vi "Seconds_to_Elapsed_Time_String.vi"(10 "# Seconds (0)":u32) -> (2 "Elapsed Time (00:00:00)":string="00:00:00")   [LabVIEW 2014, in "UI_ProgressDlg.lvlib" / "UI_ProgressDlg.lvclass"]
doc: "This VI takes an integer input of a number of seconds. It converts this to a string output of the amount of time represented in days, hours, minutes and seconds.\n\nOutput is in format\n [DD] HH:MM:SS ([days] hours:minutes:seconds)\n\nThe number of days appears only if the period # of seconds is greater than or equal to 86400, or 24 hours.\n\nThis VI was created in LabVIEW 6.1"
uses:
  UI_ProgressDlg.lvclass
panel:
  # "In LabVIEW, the time/date functions return an unsigned integer for the number of \nseconds that have elapsed since 12:00 AM Friday, January 1, 1904 Universal Time.\nThis example converts a number of seconds to a string format for a relative period of time.\n\nEnter a value for the number of seconds to convert, then run the VI.  The elapsed time \nwill be displayed according to the following format:  [days] HH:MM:SS."
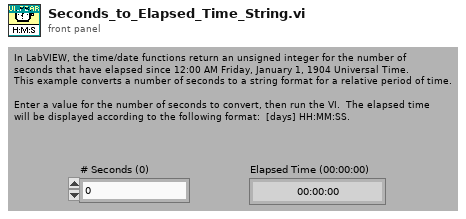
[diagram p1: front panel]
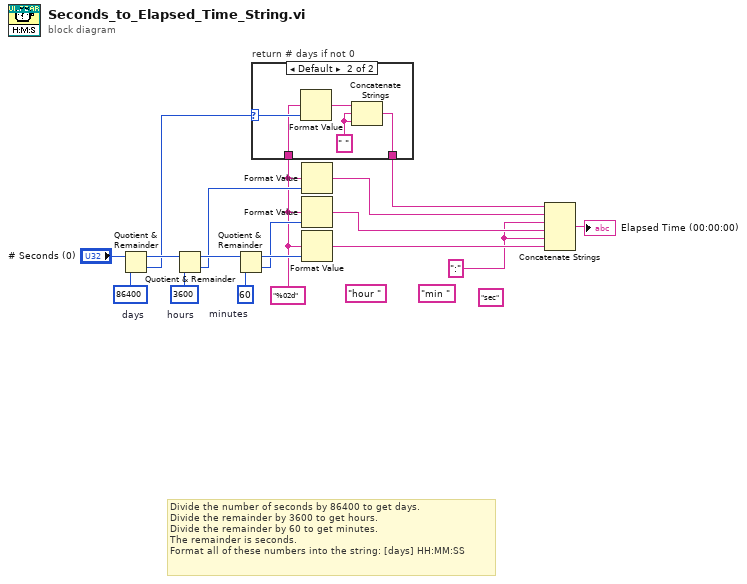
[diagram p0: block diagram]
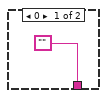
[diagram p2: hidden frame]
diagram:
  w1 = ":"
  (unwired) "sec"
  (unwired) "min "
  w5 = u32 86400  # days
  w2 = "%02d" ("format string")
  (unwired) "hour "
  w16 = u32 3600  # hours
  w15 = u32 60  # minutes
  # "Divide the number of seconds by 86400 to get days.\nDivide the remainder by 3600 to get hours.\nDivide the remainder by 60 to get minutes.\nThe remainder is seconds.\nFormat all of these numbers into the string: [days] HH:MM:SS"
  n1 = Quotient & Remainder(x="# Seconds (0)", y=w5) -> (x-y*floor(x/y)=w7:u32, floor(x/y)=w4:u32)
  n2 = Quotient & Remainder(x=w7, y=w16) -> (x-y*floor(x/y)=w17:u32, floor(x/y)=w9:u32)
  n3 = Quotient & Remainder(x=w17, y=w15) -> (x-y*floor(x/y)=w10:u32, floor(x/y)=w8:u32)
  n4 = case "return # days if not 0" shown="Default" w4 {
    selector: w4 -> [_ w23]
    tunnel: ["" w20] -> w3
    tunnel: w2 -> [_ w19]
    frame 0 {
    }
    frame Default {
      w21 = " "
      n5 = Format Value(format string=w19, value (0)=w23) -> (output string=w22:string)  [unwired: 1 in]
      n6 = Concatenate Strings(w22, w21, w21) -> (w20:string)
    }
  }
  n7 = Format Value(format string=w2, value (0)=w9) -> (output string=w11:string)  [unwired: 1 in]
  n8 = Format Value(format string=w2, value (0)=w8) -> (output string=w12:string)  [unwired: 1 in]
  n9 = Format Value(format string=w2, value (0)=w10) -> (output string=w14:string)  [unwired: 1 in]
  n10 = Concatenate Strings(w3, w11, w1, w12, w1, w14) -> (→"Elapsed Time (00:00:00)":string)
